vi "Auton2.vi"(6 "2nd Ball":bool, 8 "1st Shoot distance (ft)":dbl, 9 "Start Position":dbl, 10 "Distance from tape (ft)":dbl, 11 "2nd Shoot distance (ft)":dbl) -> ()   [LabVIEW 2013]
uses:
  <vilib>/Rock Robotics/WPI/Solenoid/WPI_SolenoidValue.ctl
  Robot Global Data.vi
  Device Refrences.vi
  <vilib>/Rock Robotics/WPI/Solenoid/WPI_SolenoidSetEnum.vi
  <vilib>/addons/control/pid/pid.llb/PID (DBL).vi
  <vilib>/addons/control/pid/NI_PID_pid.lvlib
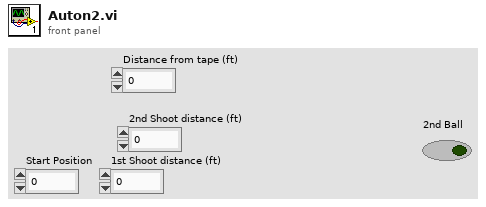
[diagram p1: front panel]
types:
  T1 = typedef "WPI_SolenoidValue.ctl" = enum16{"Off", "On", "Forward", "Reverse"}
  T2 = cluster{"proportional gain (Kc)":dbl, "integral time (Ti, min)":dbl, "derivative time (Td, min)":dbl}
  T3 = cluster{"Compressor running":bool, "Compressor enabled":bool, "Right Encoder":dbl, "Left Encoder":dbl, "Ultrasonic Sensor":dbl, "Light Sensor":dbl, "Gyro":dbl, "Left Encoder Speed":dbl, "Ball Presence":bool}
  T4 = enum16{"Simulator Robot", "Alpinista", "2014 Robot"}
  T5 = cluster{"Drive Output Values":dbl[], "Shooter Solenoid":T1, "Pickup Solenoid":T1, "Pickup Motor":dbl, "Ejecter Solenoid":T1}
  T6 = typedef "WPI_SolenoidDevRef.ctl" = cluster{"DevStatus":errorcluster, "Solenoid Module":T7, "Forward Solenoid Channel":T8, "Reverse Solenoid Channel":T8}
  T7 = typedef "FPGA_TypedefSolenoidModule.ctl" = enum16{"Solenoid Module 1", "Solenoid Module 2"}
  T8 = typedef "WPI_SolenoidChannel.ctl" = enum8{"Solenoid 1", "Solenoid 2", "Solenoid 3", "Solenoid 4", "Solenoid 5", "Solenoid 6", "Solenoid 7", "Solenoid 8", "Invalid"}
  T9 = typedef "WPI_EncoderDevRef.ctl" = cluster{"DevStatus":errorcluster, "EncoderIndex":T10, "CounterIndex":T11, "DistancePerCount":dbl, "Decoding Type":T12}
  T10 = typedef "FPGA_EncoderIdx.ctl" = enum8{"Enc 0", "Enc 1", "Enc 2", "Enc 3", "Invalid"}
  T11 = typedef "FPGA_CounterCtrSystemIndex.ctl" = enum8{"Ctr 0", "Ctr 1", "Ctr 2", "Ctr 3", "Ctr 4", "Ctr 5", "Ctr 6", "Ctr 7", "Invalid"}
  T12 = typedef "WPI_EncoderType.ctl" = enum16{"1x", "2x", "4x"}
  T13 = typedef "WPI_GyroDevRef.ctl" = cluster{"DevStatus":errorcluster, "Analog Module":T14, "Analog Channel":T15, "Offset":dbl, "Gain (VoltsPerDegree/Second)":dbl}
  T14 = typedef "FPGA_TypedefAnalogModule.ctl" = enum16{"Analog Module 1", "Analog Module 2"}
  T15 = typedef "FPGA_AIChannel.ctl" = enum8{"AI 1", "AI 2", "AI 3", "AI 4", "AI 5", "AI 6", "AI 7", "AI 8", "Invalid"}
  T16 = typedef "WPI_MotorControlDeviceRef.ctl" = cluster{"DeviceStatus":errorcluster, "Type":enum16{"PWM", "CAN"}, "PWM":cluster{"Digital Module":T17, "PWM Channel":T18, "DeadBand":T19}, "CAN":cluster{"Device Number":u8, "Control Mode":T20, "Semaphore":T21, "Max Vout":dbl}, "Invert":bool, "TransformRef":T22, "InvTransformRef":T22}
  T17 = typedef "FPGA_TypedefDigitalModule.ctl" = enum16{"Digital Module 1", "Digital Module 2"}
  T18 = typedef "FPGA_DIOPWMChannel.ctl" = enum8{"PWM 1", "PWM 2", "PWM 3", "PWM 4", "PWM 5", "PWM 6", "PWM 7", "PWM 8", "PWM 9", "PWM 10", "Invalid"}
  T19 = typedef "WPI_PWMDeadband.ctl" = cluster{"Name":string, "maxPositivePwm":i32, "minPositivePwm":i32, "centerPwm":i32, "maxNegativePwm":i32, "minNegativePwm":i32, "angularRange":u16}
  T20 = typedef "WPI_CANJaguar_ControlMode.ctl" = enum8{"Percent VBus", "Current", "Speed", "Position", "Voltage"}
  T21 = typedef "Semaphore RefNum" = refnum<k1>
  T22 = typedef "WPI_PWMTransform_ConPane.ctl" = refnum<vi>
  T23 = typedef "WPI_RobotDriveDevRef.ctl" = cluster{"DevStatus":errorcluster, "Motors[]":T16[], "Square Inputs":bool, "Max Output":dbl, "Isochronous":bool}
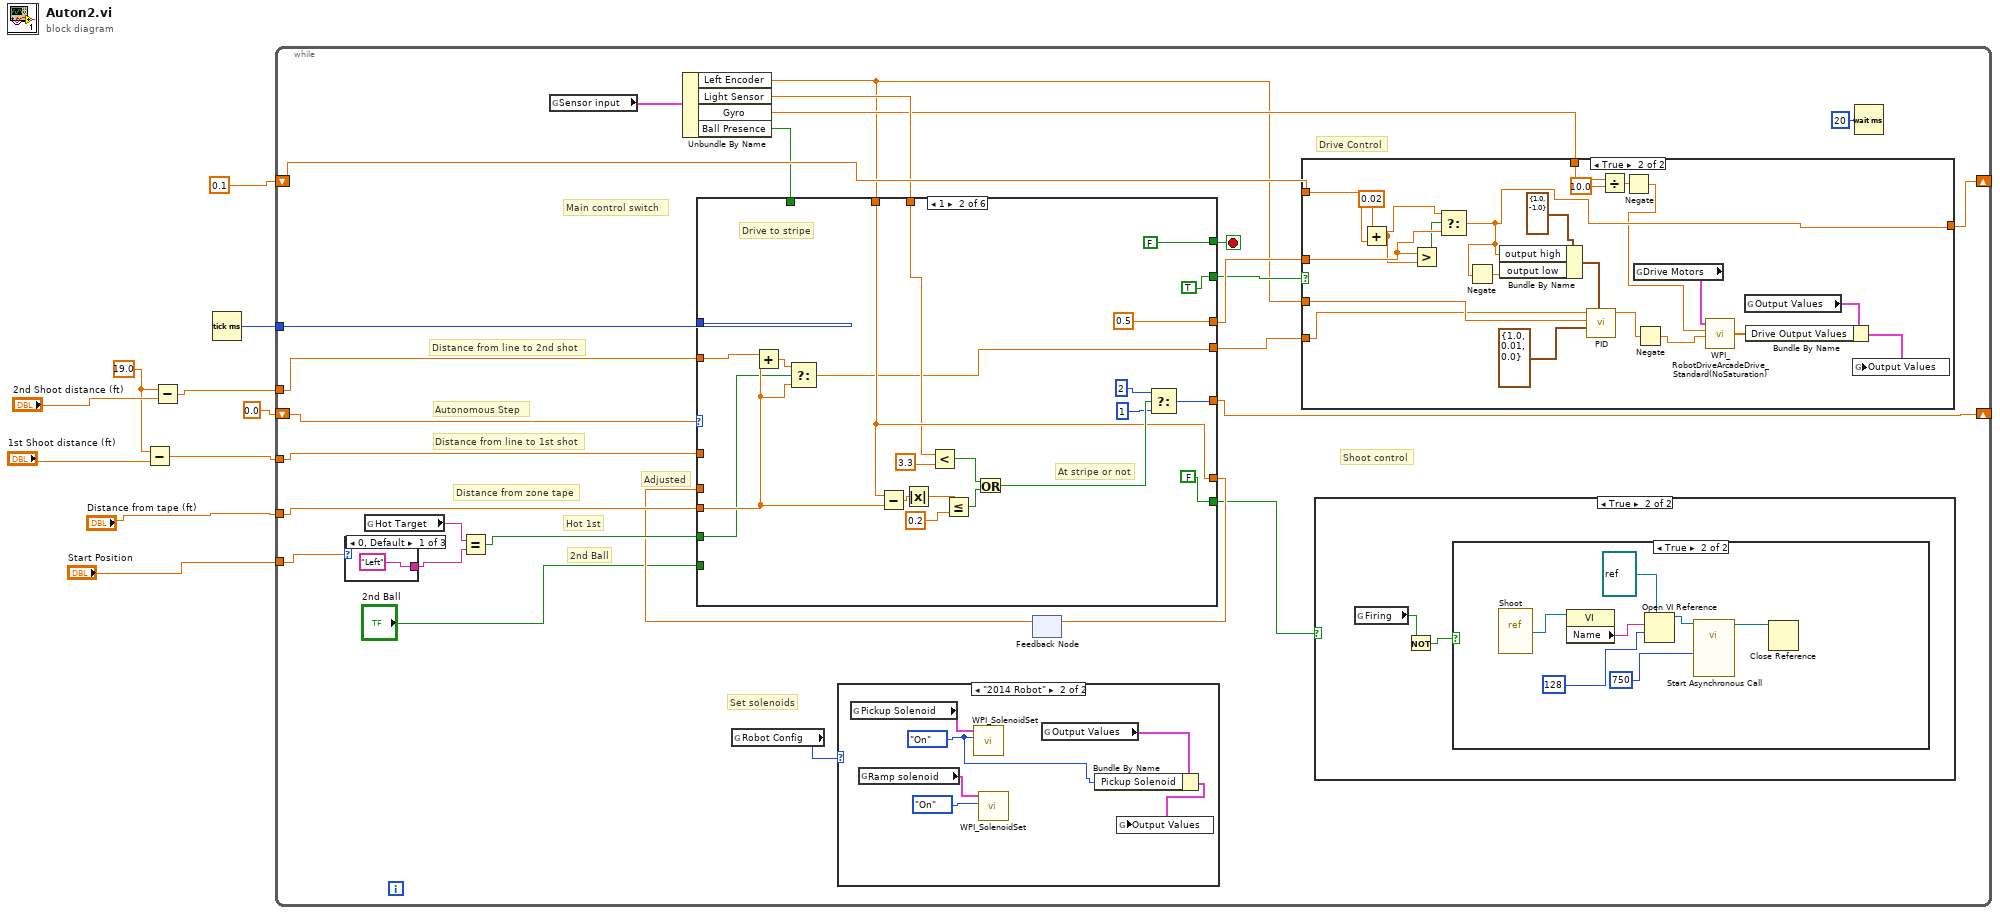
[diagram p0: block diagram]
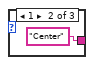
[diagram p2: hidden frame]
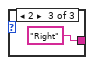
[diagram p3: hidden frame]
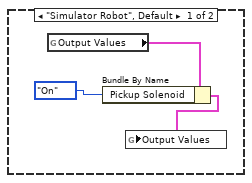
[diagram p6: hidden frame]
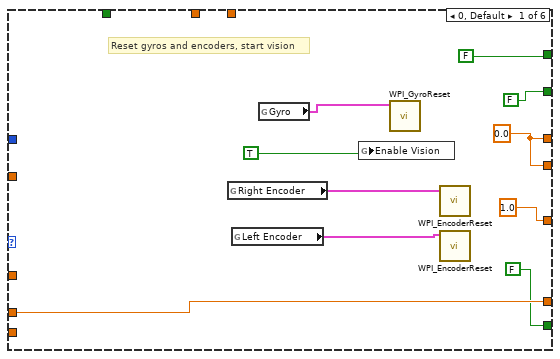
[diagram p7: hidden frame]
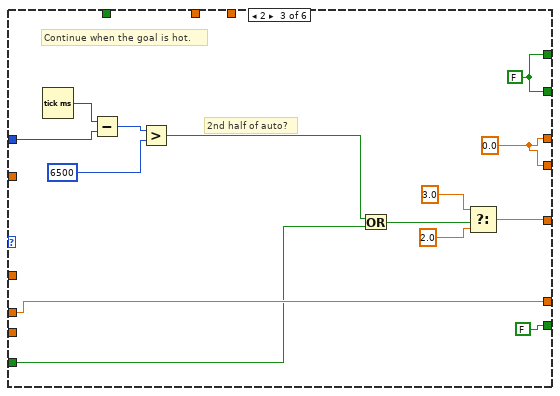
[diagram p8: hidden frame]
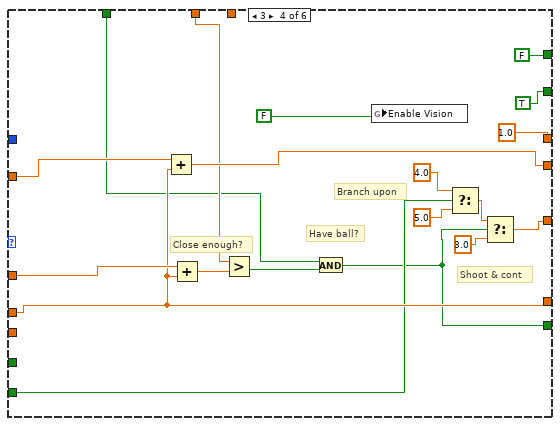
[diagram p9: hidden frame]
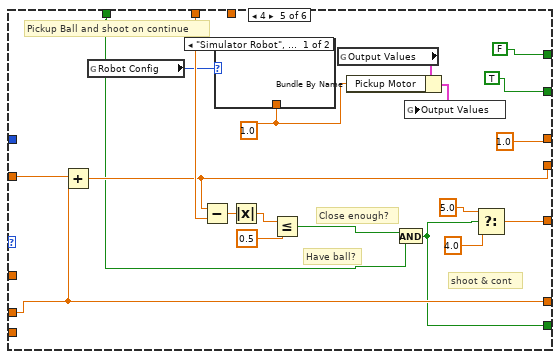
[diagram p10: hidden frame]
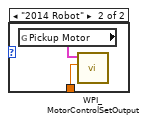
[diagram p11: hidden frame]
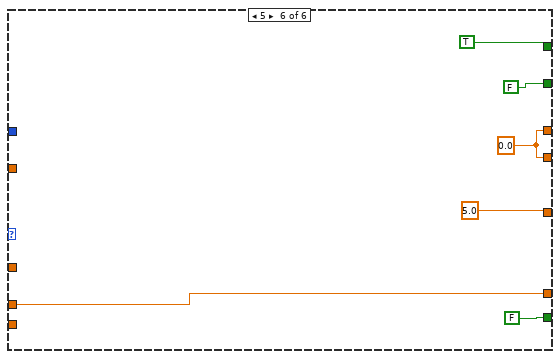
[diagram p12: hidden frame]
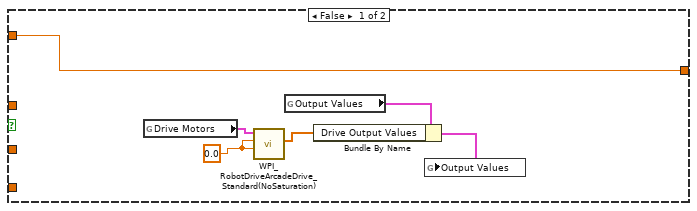
[diagram p13: hidden frame]
diagram:
  w3 = 19.0
  n1 = Subtract(x=w3, y="1st Shoot distance (ft)") -> (x-y=w1:dbl)
  n2 = Subtract(x=w3, y="2nd Shoot distance (ft)") -> (x-y=w5:dbl)
  n3 = Tick Count (ms)() -> (millisecond timer value=w7:u32)
  n4 = while {
    shift-right: [w36] -> _
    shift-left: 0.1 -> [w37]
    shift-right: [w31] -> _
    shift-left: 0.0 -> [w32]
    tunnel: w5 -> [w30]
    tunnel: "Distance from tape (ft)" -> [w19]
    tunnel: "Start Position" -> [w13]
    tunnel: w7 -> [w25]
    tunnel: w1 -> [w20]
    stop <- w21 stop-if-true
    # "Adjusted"
    # "2nd Ball"
    # "Hot 1st"
    # "Distance from zone tape"
    # "Distance from line to 1st shot"
    # "Autonomous Step"
    # "Distance from line to 2nd shot"
    # "Set solenoids"
    # "Shoot control"
    # "Drive Control"
    # "Main control switch"
    n5 = case shown="0, Default" w13 {
      tunnel: ["Left" "Center" "Right"] -> w16
      frame 0, Default {
      }
      frame 1 {
      }
      frame 2 {
      }
    }
    n6 = global read "Robot Global Data.vi" "Hot Target"() -> (w17:string)
    n7 = Equal?(x=w17, y=w16) -> (x = y?=w15:bool)
    n8 = global read "Robot Global Data.vi" "Sensor input"() -> (w35:T3)
    n9 = Unbundle By Name(w35) -> ("Left Encoder"=w18:dbl, "Light Sensor"=w28:dbl, "Gyro"=w24:dbl, "Ball Presence"=w11:bool)
    n10 = global read "Robot Global Data.vi" "Robot Config"() -> (w26:T4)
    n11 = case shown="\"2014 Robot\"" w26 {
      frame "Simulator Robot", Default {
        n12 = global read "Robot Global Data.vi" "Output Values"() -> (w52:T5)
        n13 = Bundle By Name(cluster=w52, "Pickup Solenoid"=WPI_SolenoidValue."On") -> (w51:T5)
        n14 = global write "Robot Global Data.vi" "Output Values"(w51) -> ()
      }
      frame "2014 Robot" {
        w54 = WPI_SolenoidValue."On" ("Value")
        n15 = global read "Device Refrences.vi" "Pickup Solenoid"() -> (w58:T6)
        n16 = global read "Device Refrences.vi" "Ramp solenoid"() -> (w56:T6)
        n17 = call-poly <vilib>:"WPI_SolenoidSet.vi"("Value"=w54, "SolenoidDevRef"=w58) -> ()  [unwired: 8 in, 2 out]
        n18 = call-poly <vilib>:"WPI_SolenoidSet.vi"("Value"=WPI_SolenoidValue."On", "SolenoidDevRef"=w56) -> ()  [unwired: 8 in, 2 out]
        n19 = global read "Robot Global Data.vi" "Output Values"() -> (w55:T5)
        n20 = Bundle By Name(cluster=w55, "Pickup Solenoid"=w54) -> (w53:T5)
        n21 = global write "Robot Global Data.vi" "Output Values"(w53) -> ()
      }
    }
    n22 = feedback #1() -> (w14:dbl)  [unwired: 1 in]
    n23 = case shown="1" w32 {
      tunnel: [w66 0.5 w93 1.0 1.0 w149] -> w33
      tunnel: [1.0 w84 w100 w116 w130 5.0] -> w31
      tunnel: [w66 w74 w93 w120 w128 w149] -> w29
      tunnel: w30 -> [_ w77 _ w121 w137 _]
      tunnel: w28 -> [_ w82 _ _ _ _]
      tunnel: w18 -> [_ w83 _ w109 w129 _]
      tunnel: w19 -> [_ w76 _ _ _ _]
      tunnel: [w68 w83 w103 w110 w136 w150] -> w27
      tunnel: w14 -> [w68 _ w103 w110 w136 w150]
      tunnel: w25 -> [_ _ w95 _ _ _]
      tunnel: [FALSE FALSE FALSE w104 w123 FALSE] -> w23
      tunnel: [FALSE TRUE w101 TRUE TRUE FALSE] -> w22
      tunnel: [FALSE FALSE w101 FALSE FALSE TRUE] -> w21
      tunnel: w20 -> [_ _ _ w111 _ _]
      tunnel: "2nd Ball" -> [_ _ _ w108 _ _]
      tunnel: w15 -> [_ w71 w91 _ _ _]
      tunnel: w11 -> [_ _ _ w105 w124 _]
      frame 0, Default {
        w66 = 0.0
        # "Reset gyros and encoders, start vision"
        n24 = global read "Device Refrences.vi" "Right Encoder"() -> (w65:T9)
        n25 = global read "Device Refrences.vi" "Left Encoder"() -> (w64:T9)
        n26 = global read "Device Refrences.vi" "Gyro"() -> (w62:T13)
        n27 = global write "Robot Global Data.vi" "Enable Vision"(TRUE) -> ()
        n28 = call <vilib>:"WPI_GyroReset.vi"("GyroDevRef"=w62) -> ()  [unwired: 9 in, 2 out]
        n29 = call <vilib>:"WPI_EncoderReset.vi"("EncoderDevRef"=w65) -> ()  [unwired: 9 in, 2 out]
        n30 = call <vilib>:"WPI_EncoderReset.vi"("EncoderDevRef"=w64) -> ()  [unwired: 9 in, 2 out]
      }
      frame 1 {
        # "At stripe or not"
        # "Drive to stripe"
        n31 = Add(x=w77, y=w76) -> (x+y=w75:dbl)
        n32 = Select(t=w75, s=w71, f=w76) -> (s? t:f=w74:dbl)
        n33 = Subtract(x=w83, y=w76) -> (x-y=w89:dbl)
        n34 = Absolute Value(x=w89) -> (abs(x)=w88:dbl)
        n35 = Less?(x=w82, y=3.3) -> (x < y?=w72:bool)
        n36 = Less Or Equal?(x=w88, y=0.2) -> (x <= y?=w86:bool)
        n37 = Or(x=w72, y=w86) -> (x .or. y?=w85:bool)
        n38 = Select(t=2, s=w85, f=1) -> (s? t:f=w84:i32)
      }
      frame 2 {
        w93 = 0.0
        w101 = FALSE
        # "2nd half of auto?"
        # "Continue when the goal is hot."
        n39 = Tick Count (ms)() -> (millisecond timer value=w96:u32)
        n40 = Subtract(x=w96, y=w95) -> (x-y=w94:u32)
        n41 = Greater?(x=w94, y=6500) -> (0:w92:bool)
        n42 = Or(x=w92, y=w91) -> (x .or. y?=w97:bool)
        n43 = Select(t=3.0, s=w97, f=2.0) -> (s? t:f=w100:dbl)
      }
      frame 3 {
        # "Shoot & cont"
        # "Have ball?"
        # "Close enough?"
        # "Branch upon"
        n44 = Add(x=w121, y=w110) -> (x+y=w120:dbl)
        n45 = Add(x=w111, y=w110) -> (x+y=w107:dbl)
        n46 = Greater?(x=w109, y=w107) -> (0:w106:bool)
        n47 = And(x=w105, y=w106) -> (x .and. y?=w104:bool)
        n48 = global write "Robot Global Data.vi" "Enable Vision"(FALSE) -> ()
        n49 = Select(t=4.0, s=w108, f=5.0) -> (s? t:f=w114:dbl)
        n50 = Select(t=w114, s=w104, f=3.0) -> (s? t:f=w116:dbl)
      }
      frame 4 {
        w127 = 1.0
        # "shoot & cont"
        # "Have ball?"
        # "Close enough?"
        # "Pickup Ball and shoot on continue"
        n51 = Add(x=w137, y=w136) -> (x+y=w128:dbl)
        n52 = global read "Robot Global Data.vi" "Robot Config"() -> (w126:T4)
        n53 = Subtract(x=w128, y=w129) -> (x-y=w132:dbl)
        n54 = case shown="\"Simulator Robot\", Default" w126 {
          tunnel: w127 -> [_ w143]
          frame "Simulator Robot", Default {
          }
          frame "2014 Robot" {
            n55 = global read "Device Refrences.vi" "Pickup Motor"() -> (w144:T16)
            n56 = call <vilib>:"WPI_MotorControlSetOutput.vi"("Output"=w143, "MotorControlDevRef"=w144) -> ()  [unwired: 7 in, 3 out]
          }
        }
        n57 = Absolute Value(x=w132) -> (abs(x)=w133:dbl)
        n58 = Less Or Equal?(x=w133, y=0.5) -> (x <= y?=w125:bool)
        n59 = global read "Robot Global Data.vi" "Output Values"() -> (w142:T5)
        n60 = Bundle By Name(cluster=w142, "Pickup Motor"=w127) -> (w141:T5)
        n61 = And(x=w125, y=w124) -> (x .and. y?=w123:bool)
        n62 = global write "Robot Global Data.vi" "Output Values"(w141) -> ()
        n63 = Select(t=5.0, s=w123, f=4.0) -> (s? t:f=w130:dbl)
      }
      frame 5 {
        w149 = 0.0
      }
    }
    n64 = feedback-in #1(w27) -> ()
    n65 = case shown="True" w22 {
      tunnel: w37 -> [w156 w178]
      tunnel: [w156 w177] -> w36
      tunnel: w33 -> [_ w170]
      tunnel: w18 -> [_ w169]
      tunnel: w29 -> [_ w168]
      tunnel: w24 -> [_ w160]
      frame False {
        w153 = 0.0
        n66 = global read "Device Refrences.vi" "Drive Motors"() -> (w152:T23)
        n67 = call <vilib>:"WPI_RobotDriveArcadeDrive_Standard(NoSaturation).vi"("Y axis value"=w153, "X axis value"=w153, "RobotDriveDevRef"=w152) -> ("Motor Values"=w155:dbl[])  [unwired: 1 in, 7 out]
        n68 = global read "Robot Global Data.vi" "Output Values"() -> (w154:T5)
        n69 = Bundle By Name(cluster=w154, "Drive Output Values"=w155) -> (w151:T5)
        n70 = global write "Robot Global Data.vi" "Output Values"(w151) -> ()
      }
      frame True {
        n71 = Add(x=0.02, y=w178) -> (x+y=w162:dbl)
        n72 = Greater?(x=w170, y=w162) -> (0:w163:bool)
        n73 = Select(t=w162, s=w163, f=w170) -> (s? t:f=w177:dbl)
        n74 = Negate(x=w177) -> (-x=w164:dbl)
        n75 = Bundle By Name(cluster=cluster{"output high":dbl, "output low":dbl} {"output high"=1.0, "output low"=-1.0} ("output range"), "output high"=w177, "output low"=w164) -> (w167:cluster{"output high":dbl, "output low":dbl})
        n76 = call-poly <vilib>:"PID.vi"("output range"=w167, "PID gains"=T2 {"proportional gain (Kc)"=1.0, "integral time (Ti, min)"=0.01, "derivative time (Td, min)"=0.0}, "process variable"=w169, "setpoint"=w168) -> ("output"=w172:dbl)  [unwired: 6 in, 1 out]
        n77 = Divide(x=w160, y=10.0) -> (x/y=w158:dbl)
        n78 = Negate(x=w158) -> (-x=w157:dbl)
        n79 = global read "Device Refrences.vi" "Drive Motors"() -> (w175:T23)
        n80 = Negate(x=w172) -> (-x=w171:dbl)
        n81 = call <vilib>:"WPI_RobotDriveArcadeDrive_Standard(NoSaturation).vi"("Y axis value"=w171, "X axis value"=w157, "RobotDriveDevRef"=w175) -> ("Motor Values"=w176:dbl[])  [unwired: 1 in, 7 out]
        n82 = global read "Robot Global Data.vi" "Output Values"() -> (w174:T5)
        n83 = Bundle By Name(cluster=w174, "Drive Output Values"=w176) -> (w173:T5)
        n84 = global write "Robot Global Data.vi" "Output Values"(w173) -> ()
      }
    }
    n85 = case shown="True" w23 {
      frame False {
      }
      frame True {
        n86 = global read "Robot Global Data.vi" "Firing"() -> (w41:bool)
        n87 = Not(x=w41) -> (.not. x?=w42:bool)
        n88 = case shown="True" w42 {
          frame False {
          }
          frame True {
            n89 = vi-ref "Shoot.vi"() -> (w49:refnum<vi>)
            n90 = property class="VI"(reference=w49) -> ("Name"=w48:string)  [unwired: 1 in, 2 out]
            n91 = Open VI Reference(type specifier VI Refnum (for type only)=refnum<vi> refnum, vi path=w48, options=128) -> (vi reference=w46:refnum<vi>)  [unwired: 1 in, 3 out]
            n92 = call-by-ref "Start Asynchronous Call"(reference=w46, "Duration"=750) -> (reference out=w44:refnum<vi>)  [unwired: 12 in, 1 out]
            n93 = Close Reference(reference=w44) -> ()  [unwired: 1 in, 1 out]
          }
        }
      }
    }
    n94 = Wait (ms)(milliseconds to wait=20) -> ()  [unwired: 1 out]
  }
